vi "calibrate_bemf.vi"(6 "timeout (25000ms)":i32=25000, 8 "error in (no error)":errorcluster, 9 "calibration type":u16(ring) items=["Both", "LSI", "FISF"], 10 "calibration wait time ms":u32=3000 min=3000, 11 "daemon reference in":refnum<k5>) -> (0 "error out":errorcluster, 2 "response":string, 3 "daemon reference out":refnum<k5>, 5 "command out":string="random")   [LabVIEW 2017]
doc: "<b>Command: </b>\"calibrate_bemf\"\n\n<b>Description: </b> This command will start bemf calibration.\n\n<b>Parameters: </b> calibration wait time in ms, calibration type\n____________________________________________\nDIPC 692 Daemon API 10.0.0.1\nSam Tee - Dyson Technology Ltd\nCopyright (c) 2024, Dyson Technology Ltd"
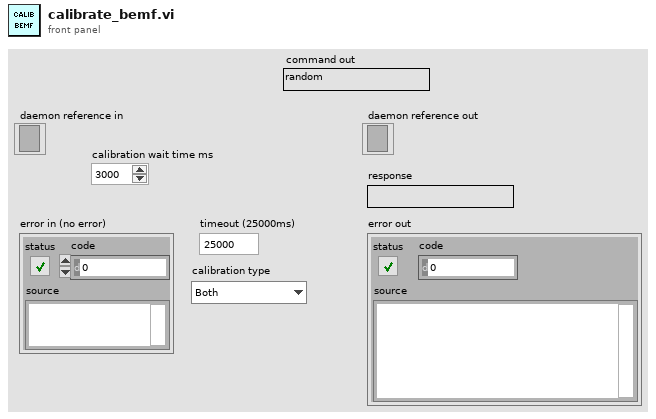
[diagram p1: front panel]
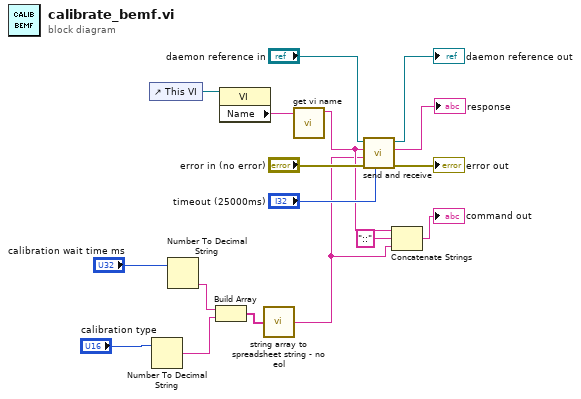
[diagram p0: block diagram]
diagram:
  n1 = control-ref of="This VI"() -> (w12:refnum<vi>)
  n2 = Number To Decimal String(number="calibration type") -> (decimal integer string=w3:string)  [unwired: 1 in]
  n3 = Number To Decimal String(number="calibration wait time ms") -> (decimal integer string=w5:string)  [unwired: 1 in]
  n4 = Build Array(w5, w3) -> (w2:string[])
  n5 = property class="VI"(reference=w12) -> ("Name"=w11:string)  [unwired: 1 in, 2 out]
  n6 = call "string array to spreadsheet string - no eol.vi"("string array"=w2) -> ("spreadsheet string - no eol"=w1:string)
  n7 = call "get vi name.vi"("library.lvlib:name.vi"=w11) -> ("vi name"=w9:string)  [unwired: 10 in]
  n8 = call "send and receive.vi"("timeout (25000ms)"="timeout (25000ms)", "error in (no error)"="error in (no error)", "data"=w1, "command"=w9, "daemon reference in"="daemon reference in") -> ("error out"=→"error out":errorcluster, "response"=→"response":string, "daemon reference out"=→"daemon reference out":refnum<k5>)  [unwired: 4 in]
  n9 = Concatenate Strings(w9, "::" ("string"), w1) -> (→"command out":string)
